vi "Save ROI Setup Files.vi"(8 "Error In":errorcluster, 10 "ROI_Information_Cluster":T2 {"Norm. XYZ Coordinates"."Apparent Frame Size" format="%#_6f"; "Norm. XYZ Coordinates"."Original FOV (um)" format="%#_6f"; "Norm. XYZ Coordinates"."Pixels per miniscan" format="%#_6f"; "Norm. XYZ Coordinates"."Dwell Time per pixel" format="%#_6f"; "Norm. XYZ Coordinates"."Resolution" format="%#_6f"; "Norm. XYZ Coordinates"."ROI group ID" format="%#_6f"; "Norm. XYZ Coordinates"."Laser Power (%)" format="%#_6f"; "Norm. XYZ Coordinates"."Zoom" format="%#_6f"; "Norm. XYZ Coordinates"."Frame Size" format="%#_6f"; "Norm. XYZ Coordinates"."Number of lines" format="%#_6f"; "Norm. XYZ Coordinates"."Composite ID" format="%#_6f"; "Norm. XYZ Coordinates"."Angle (deg)" format="%#_6f"; "Norm. XYZ Coordinates"."ROI Time (ns)" format="%#_6f"; "Norm. XYZ Coordinates"."ROI ID" format="%#_6f"; "Norm. XYZ Coordinates"."Pixels in ROI" format="%#_6f"; "Norm. XYZ Coordinates"."ROI index" format="%#_6f"; "Norm. XYZ Coordinates"."Z stop" format="%#_6f"; "Norm. XYZ Coordinates"."Y stop" format="%#_6f"; "Norm. XYZ Coordinates"."X stop" format="%#_6f"; "Norm. XYZ Coordinates"."Z start" format="%#_6f"; "Norm. XYZ Coordinates"."X start" format="%#_6f"; "Norm. XYZ Coordinates"."Y start" format="%#_6f"; "XYZ Coordinates"."Apparent Frame Size" format="%#_6f"; "XYZ Coordinates"."Original FOV (um)" format="%#_6f"; "XYZ Coordinates"."Pixels per miniscan" format="%#_6f"; "XYZ Coordinates"."Dwell Time per pixel" format="%#_6f"; "XYZ Coordinates"."Resolution" format="%#_6f"; "XYZ Coordinates"."ROI group ID" format="%#_6f"; "XYZ Coordinates"."Laser Power (%)" format="%#_6f"; "XYZ Coordinates"."Zoom" format="%#_6f"; "XYZ Coordinates"."Frame Size" format="%#_6f"; "XYZ Coordinates"."Number of lines" format="%#_6f"; "XYZ Coordinates"."Composite ID" format="%#_6f"; "XYZ Coordinates"."Angle (deg)" format="%#_6f"; "XYZ Coordinates"."ROI Time (ns)" format="%#_6f"; "XYZ Coordinates"."ROI ID" format="%#_6f"; "XYZ Coordinates"."Pixels in ROI" format="%#_6f"; "XYZ Coordinates"."ROI index" format="%#_6f"; "XYZ Coordinates"."Z stop" format="%#_6f"; "XYZ Coordinates"."Y stop" format="%#_6f"; "XYZ Coordinates"."X stop" format="%#_6f"; "XYZ Coordinates"."Z start" format="%#_6f"; "XYZ Coordinates"."X start" format="%#_6f"; "XYZ Coordinates"."Y start" format="%#_6f"}, 11 "Experiment data folder path":path) -> (0 "Error Out":errorcluster)   [LabVIEW 2020]
uses:
  Visualisation/Functional Imaging Viewer/Typedefs/ROI parameters data type.ctl
panel:
  in  "Norm. XYZ Coordinates":T1[](array[typedef]) {"Apparent Frame Size" format="%#_6f"; "Original FOV (um)" format="%#_6f"; "Pixels per miniscan" format="%#_6f"; "Dwell Time per pixel" format="%#_6f"; "Resolution" format="%#_6f"; "ROI group ID" format="%#_6f"; "Laser Power (%)" format="%#_6f"; "Zoom" format="%#_6f"; "Frame Size" format="%#_6f"; "Number of lines" format="%#_6f"; "Composite ID" format="%#_6f"; "Angle (deg)" format="%#_6f"; "ROI Time (ns)" format="%#_6f"; "ROI ID" format="%#_6f"; "Pixels in ROI" format="%#_6f"; "ROI index" format="%#_6f"; "Z stop" format="%#_6f"; "Y stop" format="%#_6f"; "X stop" format="%#_6f"; "Z start" format="%#_6f"; "X start" format="%#_6f"; "Y start" format="%#_6f"}
  out "[Z norm]":dbl[](array[numeric]) format="%#_9g"
  out "Z start":dbl format="%#_10g"
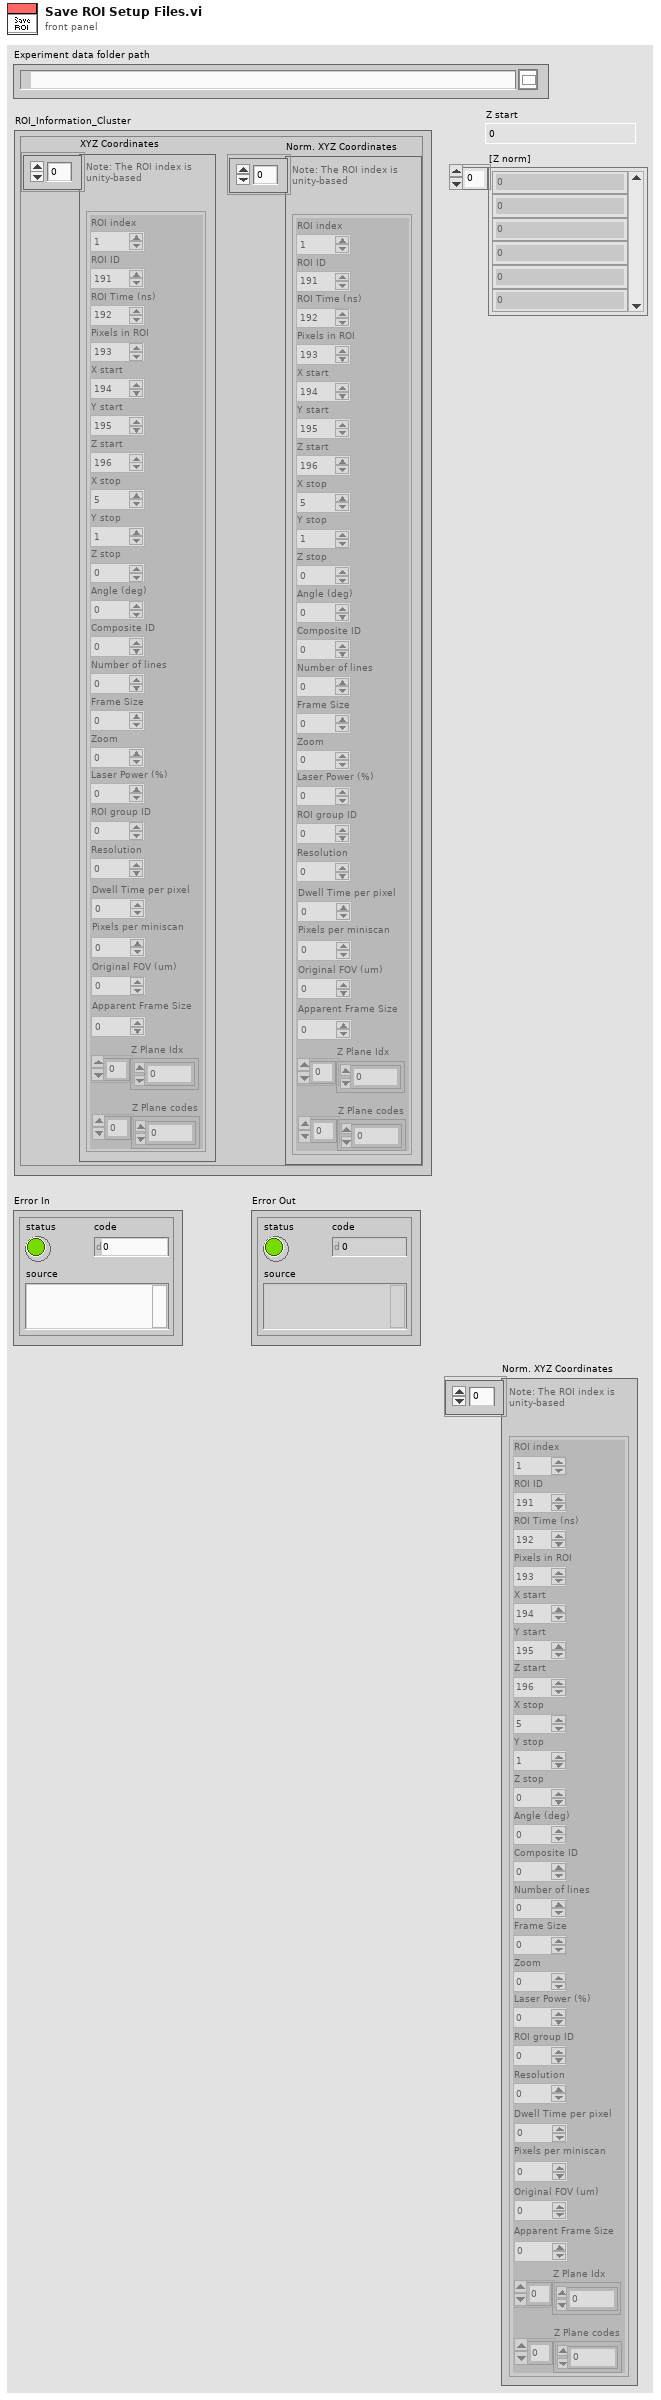
[diagram p1: front panel]
types:
  T1 = typedef "ROI parameters data type.ctl" = cluster{"ROI index":dbl, "ROI ID":dbl, "ROI Time (ns)":dbl, "Pixels in ROI":dbl, "X start":dbl, "Y start":dbl, "Z start":dbl, "X stop":dbl, "Y stop":dbl, "Z stop":dbl, "Angle (deg)":dbl, "Composite ID":dbl, "Number of lines":dbl, "Frame Size":dbl, "Zoom":dbl, "Laser Power (%)":dbl, "ROI group ID":dbl, "Resolution":dbl, "Dwell Time per pixel":dbl, "Pixels per miniscan":dbl, "Original FOV (um)":dbl, "Apparent Frame Size":dbl, "Z Plane Idx":i32[], "Z Plane codes":i32[]}
  T2 = cluster{"XYZ Coordinates":T1[], "Norm. XYZ Coordinates":T1[]}
  T3 = typedef "Fixed strings.ctl" = cluster{"ROI file name":string, "Normalised ROI file name":string, "Zplane Pockels values file name":string, "Functional data folder name":string, "Experiment Header file name":string, "Z-stack images folder name":string, "Groups setup rel. path":string, "Groups text file rel. path":string, "TDMS files folder name (F.img)":string, "TDMS files folder name (V.acq)":string, "TDMS files folder name (Pl.acq)":string, "Cycle rel times sequence file":string, "Dynamically called VIs folder name":string, "Time Series folder base name":string, "Parameter Sweep":string, "Calibration Profile Images":string}
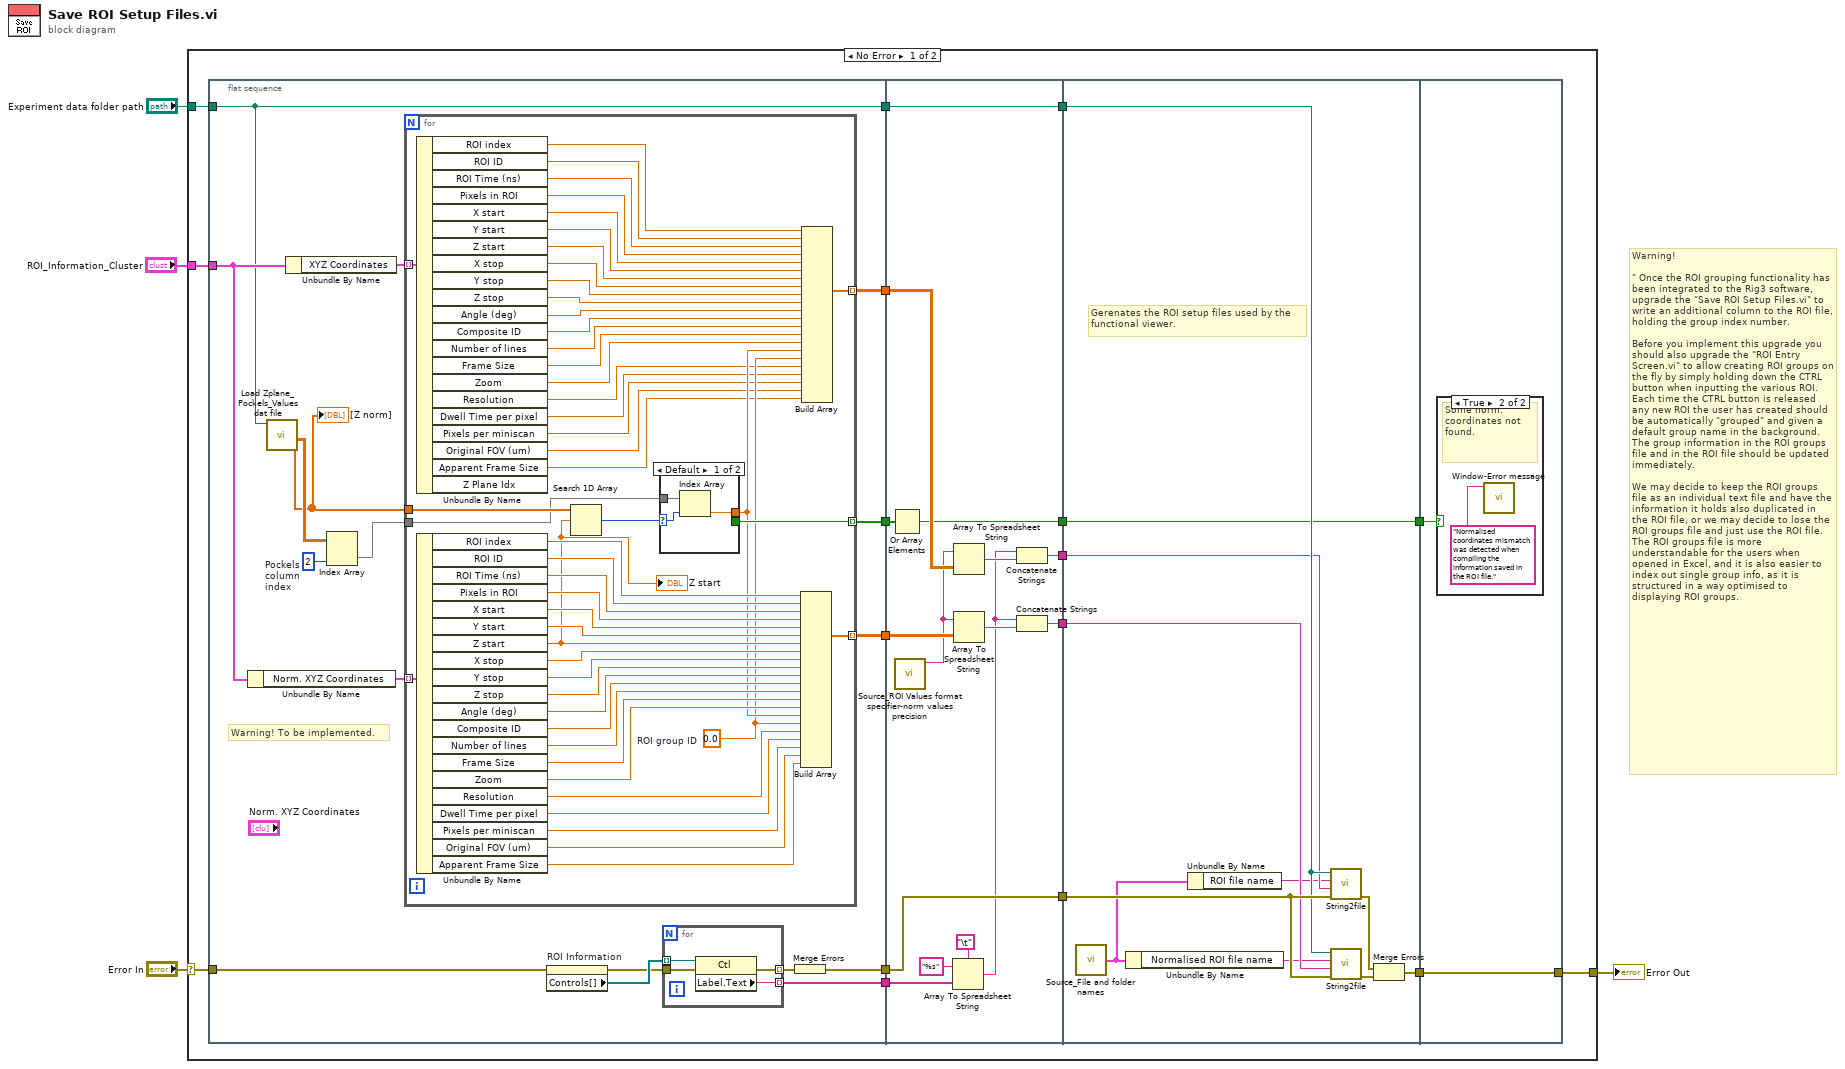
[diagram p0: block diagram]
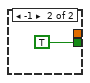
[diagram p2: hidden frame]
diagram:
  # "Warning!\n\n\"\tOnce the ROI grouping functionality has been integrated to the Rig3 software, upgrade the \"Save ROI Setup Files.vi\" to write an additional column to the ROI file, holding the group index number.\n\nBefore you implement this upgrade you should also upgrade the \"ROI Entry Screen.vi\" to allow creating ROI groups on the fly by simply holding down the CTRL button when inputting the various ROI. Each time the CTRL button is released any new ROI the user has created should be automatically \"grouped\" and given a default group name in the background. The group information in the ROI groups file and in the ROI file should be updated immediately.\n\nWe may decide to keep the ROI groups file as an individual text file and have the information it holds also duplicated in the ROI file, or we may decide to lose the ROI groups file and just use the ROI file. The ROI groups file is more understandable for the users when opened in Excel, and it is also easier to index out single group info, as it is structured in a way optimised to displaying ROI groups."
  n1 = case shown="No Error" "Error In" {
    selector: "Error In" -> [w21 w126]
    tunnel: [w14 w126] -> w3
    tunnel: "ROI_Information_Cluster" -> [w12 _]
    tunnel: "Experiment data folder path" -> [w9 _]
    frame No Error {
      n2 = flat-sequence {
        tunnel: w21 -> [w33]
        tunnel: [w22] -> w20
        tunnel: [w36] -> w19
        tunnel: [w35] -> w18
        tunnel: [w31] -> w17
        tunnel: w12 -> [w30]
        tunnel: [w26] -> w10
        tunnel: w9 -> [w26]
        tunnel: [w23] -> w8
        tunnel: w20 -> [w109]
        tunnel: w19 -> [w108]
        tunnel: w18 -> [w106]
        tunnel: w17 -> [w107]
        tunnel: [w107] -> w16
        tunnel: [w103] -> w15
        tunnel: [w102] -> w13
        tunnel: [w100] -> w11
        tunnel: w10 -> [w100]
        tunnel: w8 -> [w98]
        tunnel: [w97] -> w5
        tunnel: w16 -> [w122]
        tunnel: w15 -> [w119]
        tunnel: w13 -> [w118]
        tunnel: w11 -> [w120]
        tunnel: [w121] -> w7
        tunnel: [w112] -> w6
        tunnel: w5 -> [w112]
        tunnel: [w124] -> w14
        tunnel: w7 -> [w124]
        tunnel: w6 -> [w123]
        frame #0 {
          w28 = 2  # Pockels column index
          # "Warning! To be implemented."
          n3 = Unbundle By Name(w30) -> ("Norm. XYZ Coordinates"=w29:T1[])
          n4 = call "Load Zplane_Pockels_Values dat file.vi"("Experiment data folder path"=w26) -> ("[AOL Z (um)]"=w24:dbl[], "Zplane_Pockels_Values file data (header removed)"=w27:dbl[][])  [unwired: 5 in, 4 out]
          "[Z norm]" <- w24
          n5 = Unbundle By Name(w30) -> ("XYZ Coordinates"=w37:T1[])
          n6 = Index Array(array=w27, index (col)=w28) -> (element=w25:dbl[])  [unwired: 1 in]
          n7 = for {
            tunnel: w37 -> [w88] mode=indexing
            tunnel: w29 -> [w71] mode=indexing
            tunnel: [w70] -> w36 mode=indexing
            tunnel: [w69] -> w35 mode=indexing
            tunnel: w25 -> [w52]
            tunnel: w24 -> [w54]
            tunnel: [w51] -> w23 mode=indexing
            w49 = 0.0  # ROI group ID
            n8 = Unbundle By Name(w88) -> ("ROI index"=w87:dbl, "ROI ID"=w86:dbl, "ROI Time (ns)"=w85:dbl, "Pixels in ROI"=w84:dbl, "X start"=w83:dbl, "Y start"=w82:dbl, "Z start"=w81:dbl, "X stop"=w80:dbl, "Y stop"=w79:dbl, "Z stop"=w66:dbl, "Angle (deg)"=w67:dbl, "Composite ID"=w65:dbl, "Number of lines"=w64:dbl, "Frame Size"=w63:dbl, "Zoom"=w62:dbl, "Resolution"=w48:dbl, "Dwell Time per pixel"=w47:dbl, "Pixels per miniscan"=w44:dbl, "Original FOV (um)"=w42:dbl, "Apparent Frame Size"=w41:dbl)  [unwired: 1 out]
            n9 = Unbundle By Name(w71) -> ("ROI index"=w72:dbl, "ROI ID"=w73:dbl, "ROI Time (ns)"=w74:dbl, "Pixels in ROI"=w75:dbl, "X start"=w76:dbl, "Y start"=w56:dbl, "Z start"=w55:dbl, "X stop"=w57:dbl, "Y stop"=w77:dbl, "Z stop"=w78:dbl, "Angle (deg)"=w68:dbl, "Composite ID"=w61:dbl, "Number of lines"=w60:dbl, "Frame Size"=w59:dbl, "Zoom"=w58:dbl, "Resolution"=w46:dbl, "Dwell Time per pixel"=w45:dbl, "Pixels per miniscan"=w43:dbl, "Original FOV (um)"=w40:dbl, "Apparent Frame Size"=w39:dbl)
            "Z start" <- w55
            n10 = Search 1D Array(1D array=w54, element=w55) -> (index of element=w53:i32)  [unwired: 1 in]
            n11 = case shown="Default" w53 {
              selector: w53 -> [w90 _]
              tunnel: [_ TRUE] -> w51
              tunnel: w52 -> [w91 _]
              tunnel: [w89 _] -> w50
              frame Default {
                n12 = Index Array(array=w91, index=w90) -> (element=w89:dbl)
              }
              frame -1 {
              }
            }
            n13 = Build Array(w72, w73, w74, w75, w76, w56, w55, w57, w77, w78, w68, w61, w60, w59, w58, w50, w49, w46, w45, w43, w40, w39) -> (w69:dbl[])
            n14 = Build Array(w87, w86, w85, w84, w83, w82, w81, w80, w79, w66, w67, w65, w64, w63, w62, w50, w49, w48, w47, w44, w42, w41) -> (w70:dbl[])
          }
          n15 = property on="ROI Information" class="Clust (strict)"(error in=w33) -> (error out=w34:errorcluster, "Controls[]"=w38:refnum<vi>[])  [unwired: 1 in, 1 out]
          n16 = for {
            tunnel: w38 -> [w96] mode=indexing
            tunnel: [w95] -> w22 mode=indexing
            tunnel: [w94] -> w32 mode=indexing
            tunnel: w34 -> [w93]
            n17 = property class="Ctl"(reference=w96, error in=w93) -> (error out=w94:errorcluster, "Label.Text"=w95:string)  [unwired: 1 out]
          }
          n18 = Merge Errors(w32) -> (w31:errorcluster)
        }
        frame #1 {
          n19 = Or Array Elements(Boolean array=w98) -> (logical OR=w97:bool)
          n20 = call "Source_ROI Values format specifier-norm values precision.vi"() -> ("format (%.3f)"=w99:string)  [unwired: 11 in]
          n21 = Array To Spreadsheet String(delimiter (Tab)="\t", array=w109, 3:"%s" ("format string")) -> (spreadsheet string=w101:string)
          n22 = Array To Spreadsheet String(array=w108, 3:w99) -> (spreadsheet string=w104:string)  [unwired: 1 in]
          n23 = Array To Spreadsheet String(array=w106, 3:w99) -> (spreadsheet string=w105:string)  [unwired: 1 in]
          n24 = Concatenate Strings(w101, w104) -> (w103:string)
          n25 = Concatenate Strings(w101, w105) -> (w102:string)
        }
        frame #2 {
          # "Gerenates the ROI setup files used by the\nfunctional viewer."
          n26 = call "Source_File and folder names.vi"() -> ("Fixed strings"=w115:T3)  [unwired: 1 in]
          n27 = Unbundle By Name(w115) -> ("Normalised ROI file name"=w116:string)
          n28 = Unbundle By Name(w115) -> ("ROI file name"=w117:string)
          n29 = call "String2file.vi"("Error In"=w122, "Input String"=w119, "FileName"=w117, "Base Path"=w120) -> ("Error Out"=w114:errorcluster)  [unwired: 7 in]
          n30 = call "String2file.vi"("Error In"=w122, "Input String"=w118, "FileName"=w116, "Base Path"=w120) -> ("Error Out"=w113:errorcluster)  [unwired: 7 in]
          n31 = Merge Errors(w114, w113) -> (w121:errorcluster)
        }
        frame #3 {
          n32 = case shown="True" w123 {
            frame False {
            }
            frame True {
              # "Some norm. coordinates not found."
              n33 = call "Window-Error message.vi"("Message"="Normalised coordinates mismatch was detected when compiling the information saved in the ROI file." ("Error Source")) -> ()  [unwired: 10 in, 1 out]
            }
          }
        }
      }
    }
    frame Error {
    }
  }
  "Error Out" <- w3
